vi "XL320_VI Tree.vi"   [LabVIEW 2017, in "Dynamixel XL320.lvlib"]
doc: "This is the instrument driver for the Dynamixel Motor (RX and DX series). The VI Tree displays all the user-callable VIs of the instrument driver in an organized table."
uses:
  <instrlib>/Dynamixel XL320 (Drivers instrument)/Dynamixel XL320.lvlib
panel:
  # "Ghislain REMY, IUT de Cachan, 2015 December 2015"
  # "SEE DIAGRAM\nFOR VI TREE."
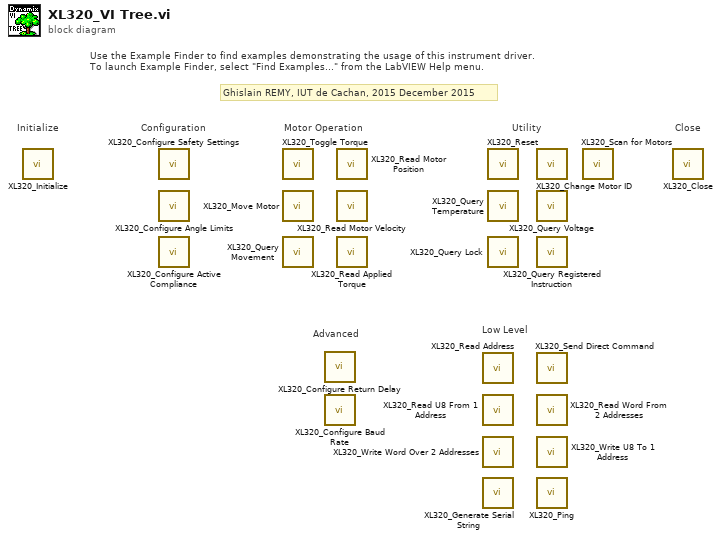
[diagram p0: block diagram]
diagram:
  # "Ghislain REMY, IUT de Cachan, 2015 December 2015"
  # "Advanced"
  # "Low Level"
  # "Use the Example Finder to find examples demonstrating the usage of this instrument driver.\nTo launch Example Finder, select \"Find Examples...\" from the LabVIEW Help menu."
  # "Configuration"
  # "Utility"
  # "Motor Operation"
  # "Close"
  # "Initialize"
  n1 = call <instrlib>:"XL320_Initialize.vi"() -> ()  [unwired: 10 in, 2 out]
  n2 = call <instrlib>:"XL320_Configure Safety Settings.vi"() -> ()  [unwired: 14 in, 2 out]
  n3 = call <instrlib>:"XL320_Configure Angle Limits.vi"() -> ()  [unwired: 14 in, 2 out]
  n4 = call <instrlib>:"XL320_Configure Active Compliance.vi"() -> ()  [unwired: 10 in, 2 out]
  n5 = call <instrlib>:"XL320_Toggle Torque.vi"() -> ()  [unwired: 10 in, 2 out]
  n6 = call <instrlib>:"XL320_Move Motor.vi"() -> ()  [unwired: 13 in, 3 out]
  n7 = call <instrlib>:"XL320_Query Movement.vi"() -> ()  [unwired: 9 in, 3 out]
  n8 = call <instrlib>:"XL320_Configure Return Delay.vi"() -> ()  [unwired: 10 in, 2 out]
  n9 = call <instrlib>:"XL320_Configure Baud Rate.vi"() -> ()  [unwired: 10 in, 2 out]
  n10 = call <instrlib>:"XL320_Read Motor Position.vi"() -> ()  [unwired: 9 in, 3 out]
  n11 = call <instrlib>:"XL320_Read Motor Velocity.vi"() -> ()  [unwired: 9 in, 3 out]
  n12 = call <instrlib>:"XL320_Read Applied Torque.vi"() -> ()  [unwired: 9 in, 3 out]
  n13 = call <instrlib>:"XL320_Read Address.vi"() -> ()  [unwired: 12 in, 4 out]
  n14 = call <instrlib>:"XL320_Read U8 From 1 Address.vi"() -> ()  [unwired: 9 in, 3 out]
  n15 = call <instrlib>:"XL320_Write Word Over 2 Addresses.vi"() -> ()  [unwired: 14 in, 2 out]
  n16 = call <instrlib>:"XL320_Generate Serial String.vi"() -> ()  [unwired: 14 in, 2 out]
  n17 = call <instrlib>:"XL320_Reset.vi"() -> ()  [unwired: 9 in, 3 out]
  n18 = call <instrlib>:"XL320_Query Temperature.vi"() -> ()  [unwired: 9 in, 3 out]
  n19 = call <instrlib>:"XL320_Query Lock.vi"() -> ()  [unwired: 9 in, 3 out]
  n20 = call <instrlib>:"XL320_Change Motor ID.vi"() -> ()  [unwired: 10 in, 2 out]
  n21 = call <instrlib>:"XL320_Query Voltage.vi"() -> ()  [unwired: 9 in, 3 out]
  n22 = call <instrlib>:"XL320_Query Registered Instruction.vi"() -> ()  [unwired: 9 in, 3 out]
  n23 = call <instrlib>:"XL320_Send Direct Command.vi"() -> ()  [unwired: 17 in, 3 out]
  n24 = call <instrlib>:"XL320_Read Word From 2 Addresses.vi"() -> ()  [unwired: 9 in, 3 out]
  n25 = call <instrlib>:"XL320_Write U8 To 1 Address.vi"() -> ()  [unwired: 14 in, 2 out]
  n26 = call <instrlib>:"XL320_Ping.vi"() -> ()  [unwired: 9 in, 3 out]
  n27 = call <instrlib>:"XL320_Scan for Motors.vi"() -> ()  [unwired: 13 in, 3 out]
  n28 = call <instrlib>:"XL320_Close.vi"() -> ()  [unwired: 11 in, 1 out]
